vi "CMN_GetHdrType.vi"(10 "keyval":string) -> (1 "type":string, 2 "keyval out":string)   [LabVIEW 2016]
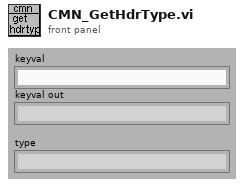
[diagram p1: front panel]
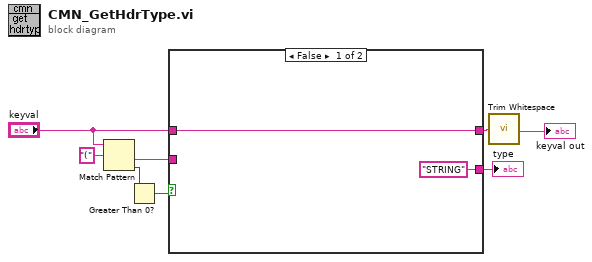
[diagram p0: block diagram]
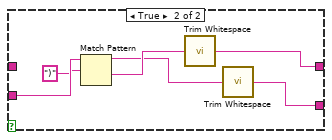
[diagram p2: hidden frame]
diagram:
  n1 = Match Pattern(string="keyval", regular expression="(") -> (after substring=w7:string, offset past match=w6:i32)  [unwired: 3 out]
  n2 = Greater Than 0?(x=w6) -> (x > 0?=w5:bool)
  n3 = case shown="False" w5 {
    tunnel: w7 -> [_ w16]
    tunnel: "keyval" -> [w10 _]
    tunnel: [w10 w14] -> w3
    tunnel: ["STRING" ("trimmed string") w13] -> w2
    frame False {
    }
    frame True {
      n4 = Match Pattern(string=w16, regular expression=")") -> (before substring=w11:string, after substring=w12:string)  [unwired: 3 out]
      n5 = call <vilib>:"Trim Whitespace.vi"("string"=w12) -> ("trimmed string"=w14:string)  [unwired: 1 in]
      n6 = call <vilib>:"Trim Whitespace.vi"("string"=w11) -> ("trimmed string"=w13:string)  [unwired: 1 in]
    }
  }
  "type" <- w2
  n7 = call <vilib>:"Trim Whitespace.vi"("string"=w3) -> ("trimmed string"=→"keyval out":string)  [unwired: 1 in]
